vi "VisionLab_Main.vi"() -> ()   [LabVIEW 2014]
uses:
  <vilib>/userdefined/High Color/IMAQdx.ctl
  <vilib>/vision/driver/NI_Vision_Acquisition_Software.lvlib
panel:
  out "whaleout":T1(plugin-control)
  in  "Color Based\nTracking?":bool=TRUE
  out "Crosshairs Display":T1(plugin-control)
  in  "Crosshairs Image Type":T2=1 items=["Grayscale (U8)", "Grayscale (I16)", "Grayscale (SGL)", "Complex (CSG)", "RGB (U32)", "HSL (U32)", "RGB (U64)", "Grayscale (U16)"]
  in  "Crosshairs Path":path=path "C:/Users/reggert/Box Sync/Olin/Year III/Robotics/RoboticsVC/Project 5 -- Vision Lab/Project/Crosshairs_Small.bmp"
  out "servo error out":errorcluster
  in  "Destination Point":cluster{"DestinationX":dbl, "DestinationY":dbl}={"DestinationX"=520.0, "DestinationY"=320.0}
  out "error out":errorcluster
  out "Live Input":T1(plugin-control)
  out "Running":bool
  in  "stop":bool
  out "FindLaser Out":T1(plugin-control)
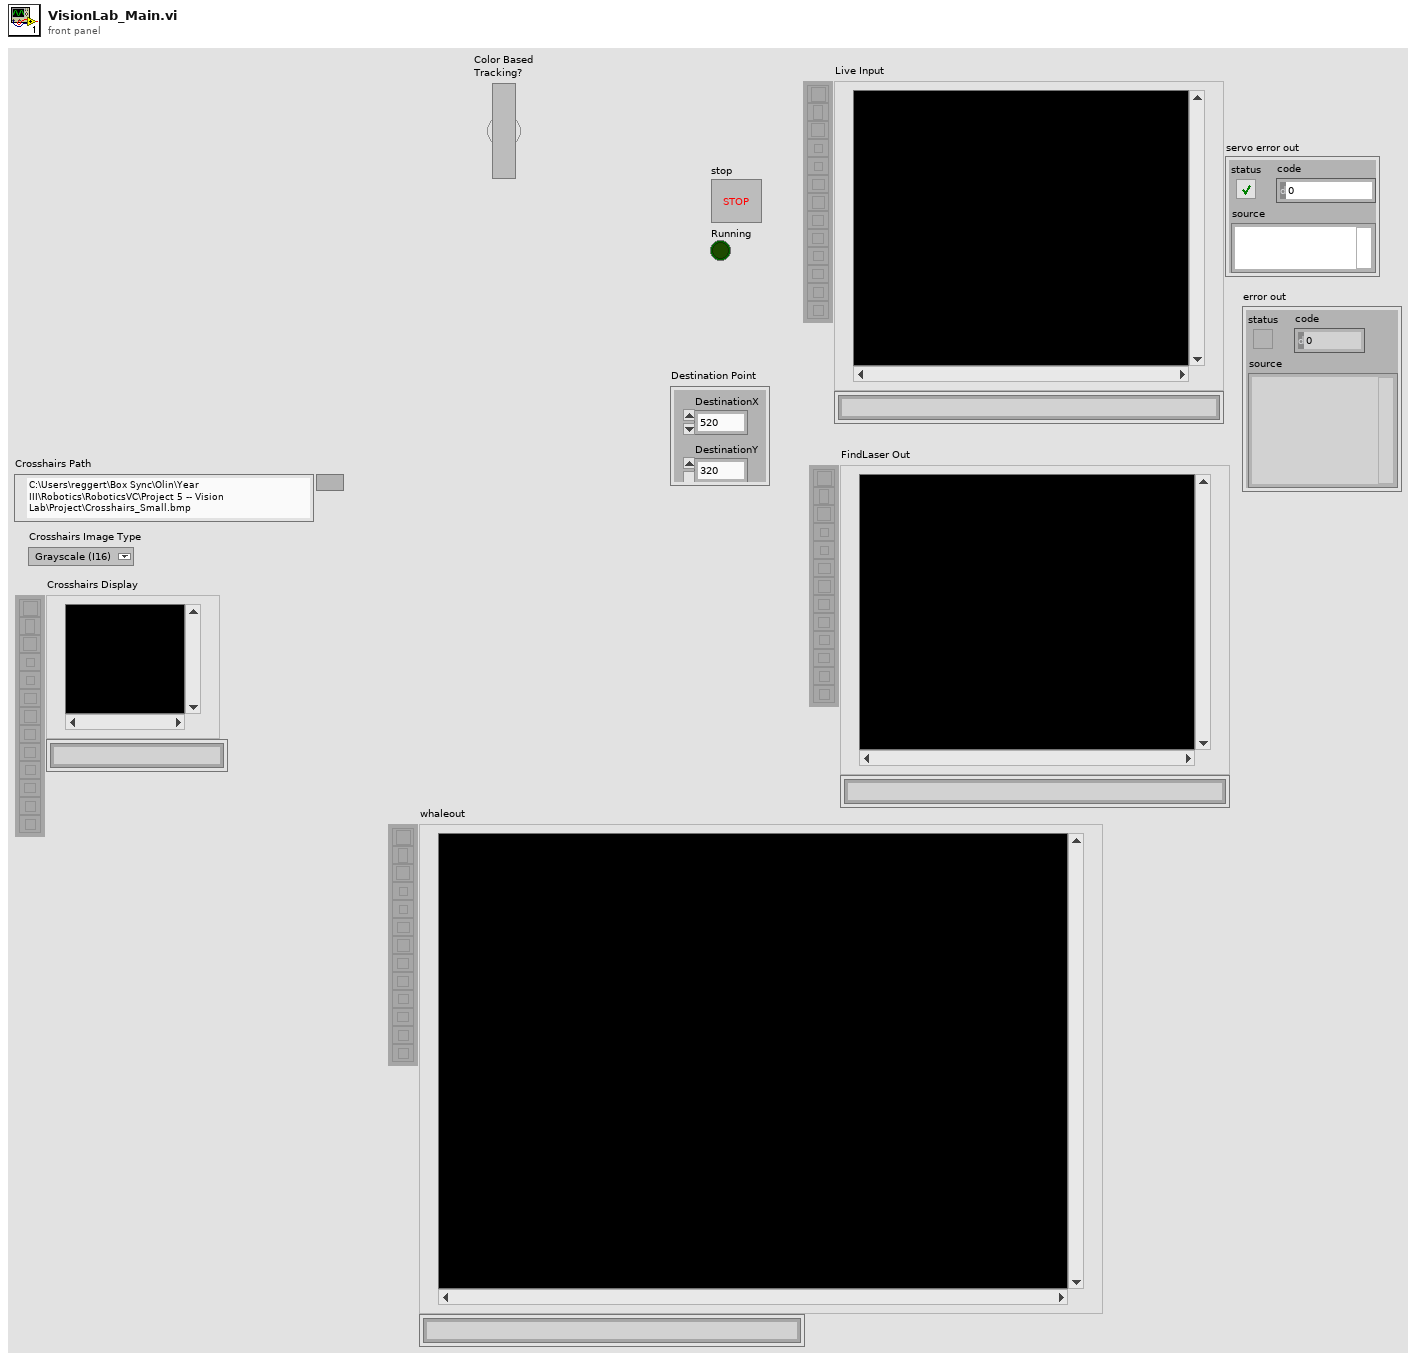
[diagram p1: front panel]
types:
  T1 = typedef "IMAQ Image.ctl" = refnum<image>
  T2 = typedef "Image Type" = u32
  T3 = typedef "IMAQdx.ctl" = refnum<k21>
  T4 = cluster{"Point1 (Pixels)":cluster{"X":sgl, "Y":sgl}, "Point2 (Pixels)":cluster{"X":sgl, "Y":sgl}, "Point1 (Real-World)":cluster{"X":sgl, "Y":sgl}, "Point2 (Real-World)":cluster{"X":sgl, "Y":sgl}, "Angle (Pixel)":dbl, "Angle (Real-World)":dbl, "Score":dbl, "Straightness":dbl, "Average SNR (db)":dbl, "Calibration Valid":bool}
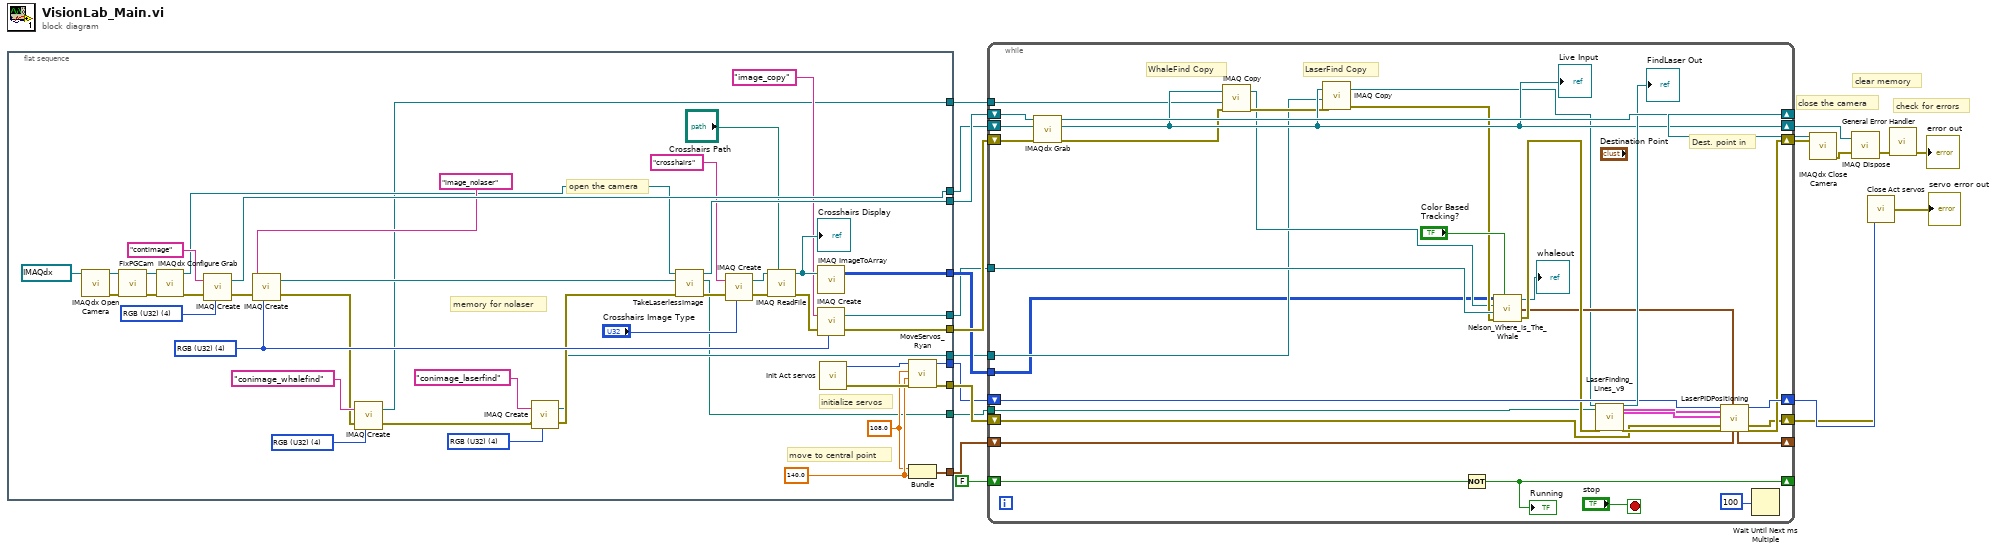
[diagram p0: block diagram]
diagram:
  # "check for errors"
  # "clear memory"
  # "close the camera"
  n1 = flat-sequence {
    tunnel: [w33] -> w21
    tunnel: [w46] -> w20
    tunnel: [w62] -> w13
    tunnel: [w55] -> w6
    tunnel: [w53] -> w9
    tunnel: [w50] -> w7
    tunnel: [w37] -> w5
    tunnel: [w32] -> w4
    tunnel: [w28] -> w3
    tunnel: [w23] -> w2
    tunnel: [w22] -> w1
    frame #0 {
      w26 = T2 4 items=["Grayscale (U8)", "Grayscale (I16)", "Grayscale (SGL)", "Complex (CSG)", "RGB (U32)", "HSL (U32)", "RGB (U64)", "Grayscale (U16)"] ("Image Type")
      w30 = T2 4 items=["Grayscale (U8)", "Grayscale (I16)", "Grayscale (SGL)", "Complex (CSG)", "RGB (U32)", "HSL (U32)", "RGB (U64)", "Grayscale (U16)"] ("Image Type")
      w35 = T2 4 items=["Grayscale (U8)", "Grayscale (I16)", "Grayscale (SGL)", "Complex (CSG)", "RGB (U32)", "HSL (U32)", "RGB (U64)", "Grayscale (U16)"] ("Image Type")
      w51 = 108.0 ("Y pos")
      w52 = 140.0 ("X pos")
      w63 = T2 4 items=["Grayscale (U8)", "Grayscale (I16)", "Grayscale (SGL)", "Complex (CSG)", "RGB (U32)", "HSL (U32)", "RGB (U64)", "Grayscale (U16)"] ("Image Type")
      # "memory for nolaser"
      # "move to central point"
      # "initialize servos"
      # "open the camera"
      n2 = call <vilib>:"IMAQdx Open Camera.vi"("Session In"=T3 "cam1") -> ("error out"=w58:errorcluster, "Session Out"=w57:T3)  [unwired: 2 in, 7 out]
      n3 = call "FixPGCam.vi"("error in"=w58, "Session In"=w57) -> ("error out"=w60:errorcluster, "IMAQdx Session Out"=w59:T3)  [unwired: 8 in]
      n4 = call <vilib>:"IMAQdx Configure Grab.vi"("error in"=w60, "Session In"=w59) -> ("error out"=w61:errorcluster, "Session Out"=w47:T3)  [unwired: 8 out]
      n5 = call "IMAQ Create"("Image Name"="contimage", "Image Type"=w63, "error in (no error)"=w61) -> ("New Image"=w62:T1, "error out"=w49:errorcluster)  [unwired: 1 in, 1 out]
      n6 = call "IMAQ Create"("Image Name"="image_nolaser", "Image Type"=w35, "error in (no error)"=w49) -> ("New Image"=w45:T1, "error out"=w29:errorcluster)  [unwired: 1 in, 1 out]
      n7 = call "IMAQ Create"("Image Name"="conimage_whalefind", "Image Type"=w30, "error in (no error)"=w29) -> ("New Image"=w28:T1, "error out"=w25:errorcluster)  [unwired: 1 in, 1 out]
      n8 = call "IMAQ Create"("Image Name"="conimage_laserfind", "Image Type"=w26, "error in (no error)"=w25) -> ("New Image"=w23:T1, "error out"=w24:errorcluster)  [unwired: 1 in, 1 out]
      n9 = call "TakeLaserlessImage.vi"("error in"=w24, "Image In"=w45, "Session In"=w47) -> ("error out"=w38:errorcluster, "nolaser Filepath"=w22:path, "Session Out"=w46:T3)  [unwired: 6 in]
      n10 = call "IMAQ Create"("Image Name"="crosshairs", "Image Type"="Crosshairs Image Type", "error in (no error)"=w38) -> ("New Image"=w44:T1, "error out"=w43:errorcluster)  [unwired: 2 in]
      n11 = call "IMAQ ReadFile"("File Path"="Crosshairs Path", "error in (no error)"=w43, "Image"=w44) -> ("error out"=w34:errorcluster, "Image Out"=w39:T1)  [unwired: 4 in, 3 out]
      "Crosshairs Display" <- w39
      n12 = call "IMAQ ImageToArray"("Image"=w39) -> ("Image Pixels (I16)"=w37:i16[][])  [unwired: 3 in, 4 out]
      n13 = call "IMAQ Create"("Image Name"="image_copy", "Image Type"=w35, "error in (no error)"=w34) -> ("New Image"=w32:T1, "error out"=w33:errorcluster)  [unwired: 2 in]
      n14 = call "Init Act servos.vi"() -> ("Device Out"=w56:i32, "error out"=w54:errorcluster)  [unwired: 1 in, 1 out]
      n15 = call "MoveServos_Ryan.vi"("servo error in"=w54, "Y pos"=w52, "X pos"=w51, "Device In"=w56) -> ("servo error out"=w53:errorcluster, "Device Out"=w55:i32)  [unwired: 6 in]
      n16 = Bundle("Y pos"=w51, "X pos"=w52) -> (w50:cluster{"Y pos":dbl, "X pos":dbl})  [unwired: 1 in]
    }
  }
  n17 = while {
    shift-right: [w96] -> w19
    shift-left: w20 -> [w98]
    shift-right: [w75] -> w17
    shift-left: w13 -> [w91]
    shift-right: [w85] -> w11
    shift-left: w21 -> [w97]
    shift-right: [w94] -> _
    shift-left: FALSE -> [w95]
    shift-right: [w88] -> w12
    shift-left: w6 -> [w81]
    shift-right: [w87] -> _
    shift-left: w7 -> [w86]
    shift-right: [w82] -> w8
    shift-left: w9 -> [w83]
    tunnel: w5 -> [w67]
    tunnel: w4 -> [w80]
    tunnel: w3 -> [w70]
    tunnel: w2 -> [w69]
    tunnel: w1 -> [w66]
    stop <- "stop" stop-if-true
    # "LaserFind Copy"
    # "WhaleFind Copy"
    # "Dest. point in"
    n18 = call <vilib>:"IMAQdx Grab.vi"("error in"=w97, "Image In"=w91, "Session In"=w98) -> ("error out"=w73:errorcluster, "Image Out"=w75:T1, "Session Out"=w96:T3)  [unwired: 1 in, 5 out]
    "Live Input" <- w75
    n19 = call "IMAQ Copy"("error in (no error)"=w73, "Image Dst"=w70, "Image Src"=w75) -> ("error out"=w74:errorcluster, "Image Dst Out"=w71:T1)  [unwired: 3 in]
    n20 = call "IMAQ Copy"("error in (no error)"=w74, "Image Dst"=w69, "Image Src"=w75) -> ("error out"=w72:errorcluster, "Image Dst Out"=w68:T1)  [unwired: 3 in]
    n21 = Not(x=w95) -> (.not. x?=w94:bool)
    "Running" <- w94
    n22 = call "Nelson_Where_is_The_Whale.vi"("Crosshair Bitmap"=w67, "Image In"=w71, "Image Copy"=w80, "error in"=w72, "Color Based\nTracking?"="Color Based\nTracking?") -> ("Image"=→"whaleout":T1, "Whale Position"=w78:cluster{"Y":dbl, "X":dbl}, "error out"=w79:errorcluster)
    n23 = call "LaserFinding_Lines_v9.vi"("Image In"=w68, "File Path (Get Image without Laser)"=w66, "error in"=w79) -> ("Image Out"=→"FindLaser Out":T1, "Straight Edge (Find Vert. Edge)"=w89:T4, "Straight Edge (Find Horiz. Edge)"=w90:T4, "error out"=w84:errorcluster)  [unwired: 21 in]
    n24 = call "LaserPIDPositioning.vi"("Servo Device In"=w81, "Vertical Edge"=w89, "Horizontal Edge"=w90, "servo error in"=w83, "error in"=w84, "Destination Point"=w78, "Servo Angles In"=w86) -> ("Servo Angles Out"=w87:cluster{"Angle X":dbl, "Angle Y":dbl}, "Servo Device Out"=w88:i32, "servo error out"=w82:errorcluster, "error out"=w85:errorcluster)  [unwired: 9 in]
    n25 = Wait Until Next ms Multiple(millisecond multiple=u32 100 ("milliseconds to wait")) -> ()  [unwired: 1 out]
  }
  n26 = call <vilib>:"IMAQdx Close Camera.vi"("error in"=w11, "Session In"=w19) -> ("error out"=w18:errorcluster)  [unwired: 9 out]
  n27 = call "IMAQ Dispose"("Image"=w17, "error in (no error)"=w18) -> ("error out"=w16:errorcluster)  [unwired: 1 in, 3 out]
  n28 = call "Close Act servos.vi"("error in"=w8, "Device In"=w12) -> ("error out"=→"servo error out":errorcluster)
  n29 = call <vilib>:"General Error Handler.vi"("error in (no error)"=w16) -> ("error out"=→"error out":errorcluster)  [unwired: 2 in, 12 out]
